vi "Forward Data.vi"(8 "error in (no error)":errorcluster, 10 "Data":T1, 11 "Data Processor Module in":refnum<class "Data Processor Module.lvclass">) -> (0 "error out":errorcluster, 2 "Data dup":T1, 3 "Data Processor Module out":refnum<class "Data Processor Module.lvclass">)   [LabVIEW 2020, in "VolatusData.lvlib" / "Data Processor Module.lvclass"]
uses:
  Data Processor Module.lvclass
  Data Processor Module.lvclass/Data Processor Module.ctl
  Forwarded Data.ctl
  VolatusData.lvlib
  Volatus/MessageQ/MessageQ.lvclass
  New Data.ctl
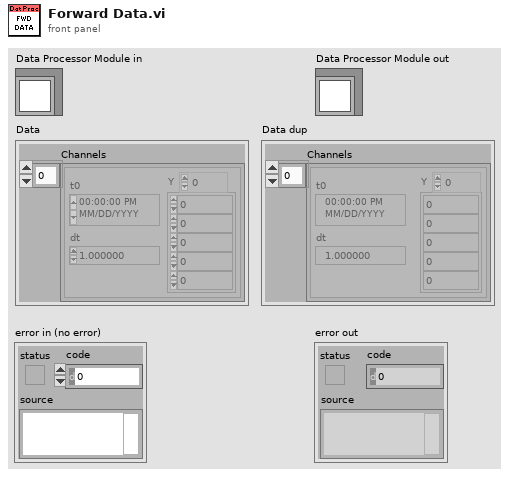
[diagram p1: front panel]
types:
  T1 = typedef "VolatusData.lvlib/New Data.ctl" = cluster{"Channels":waveform(dbl)[]}
  T2 = typedef "VolatusData.lvlib/Forwarded Data.ctl" = cluster{"Group":string, "Channels":waveform(dbl)[]}
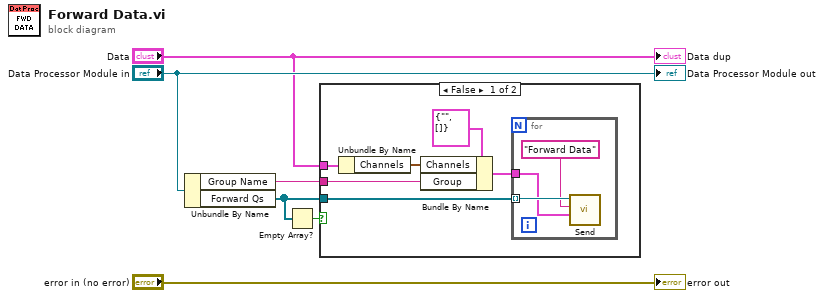
[diagram p0: block diagram]
diagram:
  n1 = Unbundle By Name("Data Processor Module in") -> ("Group Name"=w2:string, "Forward Qs"=w3:refnum<class "MessageQ.lvclass">[])
  n2 = Empty Array?(array=w3) -> (empty?=w4:bool)
  n3 = case shown="False" w4 {
    tunnel: w3 -> [w7 _]
    tunnel: w2 -> [w11 _]
    tunnel: "Data" -> [w10 _]
    frame False {
      n4 = Unbundle By Name(w10) -> ("Channels"=w9:waveform(dbl)[])
      n5 = Bundle By Name(cluster=T2 {"Group"="", "Channels"=[]} ("Forwarded Data"), "Channels"=w9, "Group"=w11) -> (w8:T2)
      n6 = for {
        tunnel: w8 -> [w13]
        tunnel: w7 -> [w15] mode=indexing
        n7 = call "Send.vi"("Data"=w13, "ID"="Forward Data", "MessageQ in"=w15) -> ()  [unwired: 7 in, 2 out]
      }
    }
    frame True {
    }
  }
  "error out" <- "error in (no error)"
  "Data Processor Module out" <- "Data Processor Module in"
  "Data dup" <- "Data"
